vi "OAT State Machine Generate Events for Numerics.vi"(1 "Initialize":bool, 2 "Numerics":dbl[](array[numeric]) format="%.2f", 4 "Event":T1(array[ring])) -> (7 "Event Found?":bool[](array[boolean]))   [LabVIEW 2017]
doc: "Detects events for the numeric objects. The event of numeric range from changed, zero crossing,sign reversed and so on. When the event detected, the coresponding output is TRUE."
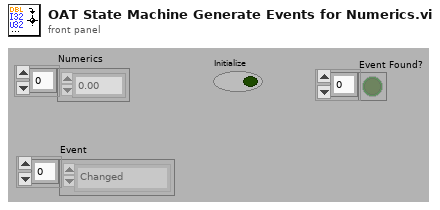
[diagram p1: front panel]
types:
  T1 = enum16{"Changed", ">0 to <0", "<0 to >0", ">0 to <=0", "<=0 to >0", ">=0 to <0", "<0 to >=0", ">0 to =0", "=0 to >0", "<0 to =0", "=0 to <0", "=0", "Zero Crossing", "Sign Reversed"}[]
  T2 = enum16{"Changed", ">0 to <0", "<0 to >0", ">0 to <=0", "<=0 to >0", ">=0 to <0", "<0 to >=0", ">0 to =0", "=0 to >0", "<0 to =0", "=0 to <0", "=0", "Zero Crossing", "Sign Reversed"}
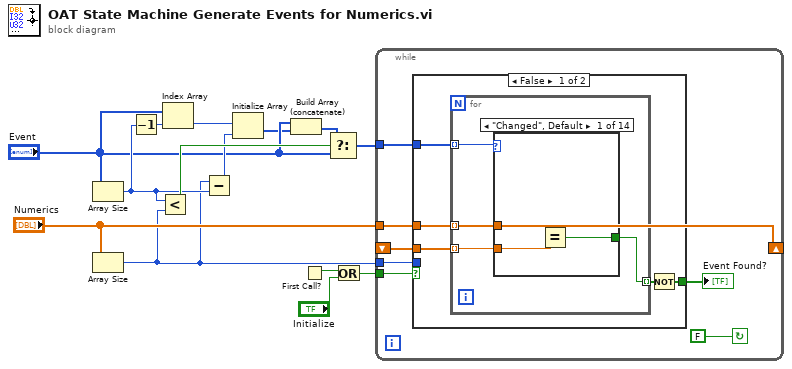
[diagram p0: block diagram]
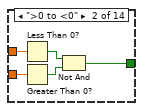
[diagram p2: hidden frame]
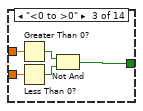
[diagram p3: hidden frame]
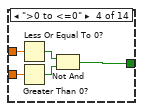
[diagram p4: hidden frame]
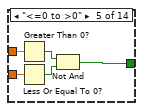
[diagram p5: hidden frame]
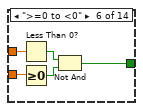
[diagram p6: hidden frame]
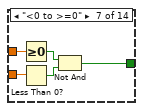
[diagram p7: hidden frame]
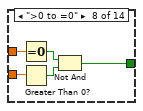
[diagram p8: hidden frame]
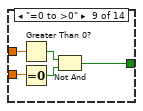
[diagram p9: hidden frame]
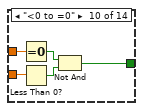
[diagram p10: hidden frame]
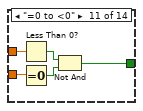
[diagram p11: hidden frame]
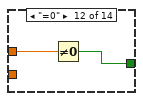
[diagram p12: hidden frame]
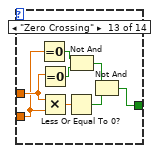
[diagram p13: hidden frame]
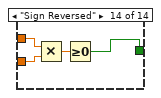
[diagram p14: hidden frame]
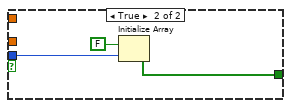
[diagram p15: hidden frame]
diagram:
  n1 = Array Size(array="Event") -> (size(s)=w9:i32)
  n2 = Array Size(array="Numerics") -> (size(s)=w4:i32)
  n3 = Decrement(x=w9) -> (x-1=w10:i32)
  n4 = Less?(x=w9, y=w4) -> (x < y?=w11:bool)
  n5 = Index Array(array="Event", index=w10) -> (element=w13:T2)
  n6 = Subtract(x=w4, y=w9) -> (x-y=w8:i32)
  n7 = Initialize Array(w13, w8) -> (w5:T1)
  n8 = Build Array (concatenate)("Event", w5) -> (w7:T1)
  n9 = First Call?() -> (First Call?: T/F=w2:bool)
  n10 = Select(t=w7, s=w11, f="Event") -> (s? t:f=w12:T1)
  n11 = Or(x=w2, y="Initialize") -> (x .or. y?=w3:bool)
  n12 = while {
    tunnel: w4 -> [w15]
    tunnel: w3 -> [w16]
    tunnel: "Numerics" -> [w19]
    shift-left: _ -> [w20]
    shift-right: [w19] -> _
    tunnel: w12 -> [w21]
    stop <- FALSE continue-if-true
    n13 = case shown="False" w16 {
      tunnel: w21 -> [w26 _]
      tunnel: w20 -> [w25 _]
      tunnel: w19 -> [w24 _]
      tunnel: [w22 w98] -> w17
      tunnel: w15 -> [_ w100]
      frame False {
        n14 = for {
          tunnel: w26 -> [w30] mode=indexing
          tunnel: w25 -> [w28] mode=indexing
          tunnel: w24 -> [w29] mode=indexing
          tunnel: [w27] -> w23 mode=indexing
          n15 = case shown="\"Changed\", Default" w30 {
            tunnel: w29 -> [w33 w38 w43 w48 w53 w57 w62 w67 w72 w77 w82 w85 w92 w96]
            tunnel: w28 -> [w32 w37 w42 w47 w52 w58 w63 w68 w73 w78 w83 _ w91 w97]
            tunnel: [w31 w34 w39 w44 w49 w54 w59 w64 w69 w74 w79 w84 w88 w94] -> w27
            frame "Changed", Default {
              n16 = Equal?(x=w33, y=w32) -> (x = y?=w31:bool)
            }
            frame ">0 to <0" {
              n17 = Less Than 0?(x=w38) -> (x < 0?=w35:bool)
              n18 = Greater Than 0?(x=w37) -> (x > 0?=w36:bool)
              n19 = Not And(1:w36, 2:w35) -> (0:w34:bool)
            }
            frame "<0 to >0" {
              n20 = Greater Than 0?(x=w43) -> (x > 0?=w41:bool)
              n21 = Less Than 0?(x=w42) -> (x < 0?=w40:bool)
              n22 = Not And(1:w40, 2:w41) -> (0:w39:bool)
            }
            frame ">0 to <=0" {
              n23 = Less Or Equal To 0?(x=w48) -> (x <= 0?=w46:bool)
              n24 = Greater Than 0?(x=w47) -> (x > 0?=w45:bool)
              n25 = Not And(1:w45, 2:w46) -> (0:w44:bool)
            }
            frame "<=0 to >0" {
              n26 = Greater Than 0?(x=w53) -> (x > 0?=w51:bool)
              n27 = Less Or Equal To 0?(x=w52) -> (x <= 0?=w50:bool)
              n28 = Not And(1:w50, 2:w51) -> (0:w49:bool)
            }
            frame ">=0 to <0" {
              n29 = Less Than 0?(x=w57) -> (x < 0?=w56:bool)
              n30 = Greater Or Equal To 0?(x=w58) -> (x >= 0?=w55:bool)
              n31 = Not And(1:w55, 2:w56) -> (0:w54:bool)
            }
            frame "<0 to >=0" {
              n32 = Greater Or Equal To 0?(x=w62) -> (x >= 0?=w61:bool)
              n33 = Less Than 0?(x=w63) -> (x < 0?=w60:bool)
              n34 = Not And(1:w60, 2:w61) -> (0:w59:bool)
            }
            frame ">0 to =0" {
              n35 = Equal To 0?(x=w67) -> (x = 0?=w66:bool)
              n36 = Greater Than 0?(x=w68) -> (x > 0?=w65:bool)
              n37 = Not And(1:w65, 2:w66) -> (0:w64:bool)
            }
            frame "=0 to >0" {
              n38 = Greater Than 0?(x=w72) -> (x > 0?=w71:bool)
              n39 = Equal To 0?(x=w73) -> (x = 0?=w70:bool)
              n40 = Not And(1:w70, 2:w71) -> (0:w69:bool)
            }
            frame "<0 to =0" {
              n41 = Equal To 0?(x=w77) -> (x = 0?=w76:bool)
              n42 = Less Than 0?(x=w78) -> (x < 0?=w75:bool)
              n43 = Not And(1:w75, 2:w76) -> (0:w74:bool)
            }
            frame "=0 to <0" {
              n44 = Less Than 0?(x=w82) -> (x < 0?=w81:bool)
              n45 = Equal To 0?(x=w83) -> (x = 0?=w80:bool)
              n46 = Not And(1:w80, 2:w81) -> (0:w79:bool)
            }
            frame "=0" {
              n47 = Not Equal To 0?(x=w85) -> (x != 0?=w84:bool)
            }
            frame "Zero Crossing" {
              n48 = Equal To 0?(x=w91) -> (x = 0?=w89:bool)
              n49 = Equal To 0?(x=w92) -> (x = 0?=w90:bool)
              n50 = Multiply(x=w92, y=w91) -> (x*y=w93:dbl)
              n51 = Less Or Equal To 0?(x=w93) -> (x <= 0?=w86:bool)
              n52 = Not And(1:w90, 2:w89) -> (0:w87:bool)
              n53 = Not And(1:w86, 2:w87) -> (0:w88:bool)
            }
            frame "Sign Reversed" {
              n54 = Multiply(x=w96, y=w97) -> (x*y=w95:dbl)
              n55 = Greater Or Equal To 0?(x=w95) -> (x >= 0?=w94:bool)
            }
          }
        }
        n56 = Not(x=w23) -> (.not. x?=w22:bool[])
      }
      frame True {
        n57 = Initialize Array(FALSE, w100) -> (w98:bool[])
      }
    }
    "Event Found?" <- w17
  }
